vi "oa_Decimation with CIC Filter (Split States).vi"(0 "x[n]":dbl[](array[numeric]) format="%.2f", 1 "reset? (True)":bool=TRUE, 5 "CIC decimation setting":T1, 9 "CIC state":dbl[](array[numeric]), 11 "error in (no error)":errorcluster, 13 "interpolation factor":i32) -> (4 "x[n] out":dbl[](array[numeric]) format="%.2f", 10 "final CIC state":dbl[](array[numeric]), 15 "error out":errorcluster)   [LabVIEW 2017, in "SoundVib_Resampling.lvlib"]
uses:
  <vilib>/addons/Sound and Vibration/Order Analysis/Resample Order Tracking/SoundVib_Resampling.lvlib
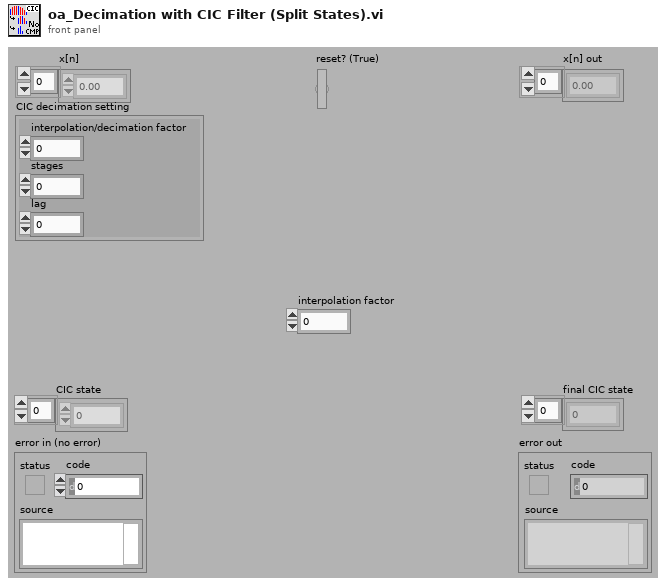
[diagram p1: front panel]
types:
  T1 = cluster{"interpolation/decimation factor":i32, "stages":i32, "lag":i32}
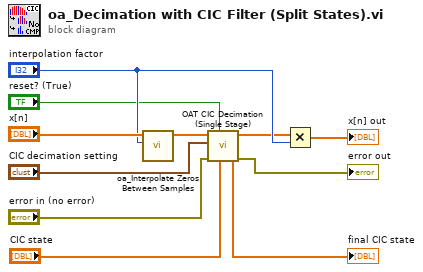
[diagram p0: block diagram]
diagram:
  n1 = call <vilib>:"oa_Interpolate Zeros Between Samples.vi"("interpolation factor"="interpolation factor", "x"="x[n]") -> ("x out"=w7:dbl[])  [unwired: 9 in]
  n2 = call <vilib>:"OAT CIC Decimation (Single Stage).vi"("initial state"="CIC state", "reset? (True)"="reset? (True)", "error in (no error)"="error in (no error)", "CIC filter settings"="CIC decimation setting", "X"=w7) -> ("error out"=→"error out":errorcluster, "Y"=w2:dbl[], "final state"=→"final CIC state":dbl[])  [unwired: 4 in]
  n3 = Multiply(x=w2, y="interpolation factor") -> (x*y=→"x[n] out":dbl[])
